vi "HS_EnableFrameBuffer.vi"(8 "error in":errorcluster, 9 "Console In":string, 11 "VISA Refnum in":refnum<visa-resource-name>) -> (0 "error out":errorcluster, 1 "Console Out":string, 2 "Reply":string, 3 "VISA Refnum out":refnum<visa-resource-name>)   [LabVIEW 2016]
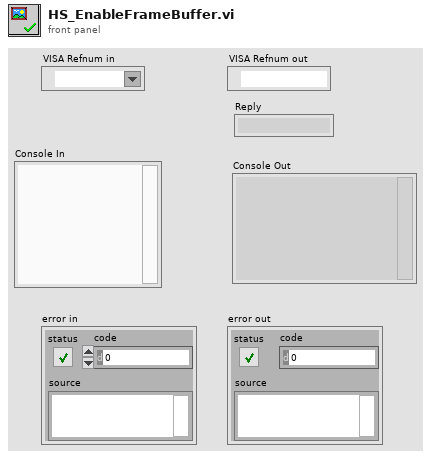
[diagram p1: front panel]
types:
  T1 = cluster{"Before":u8, "After":u8, "Send as 1 block?":bool}
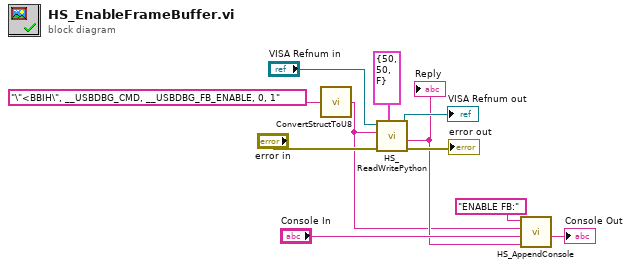
[diagram p0: block diagram]
diagram:
  n1 = call "ConvertStructToU8.vi"("struct"="\"<BBIH\", __USBDBG_CMD, __USBDBG_FB_ENABLE, 0, 1" ("write buffer")) -> ("Binary"=w2:string)
  n2 = call "HS_ReadWritePython.vi"("Timeouts (ms)"=T1 {"Before"=50, "After"=50, "Send as 1 block?"=FALSE}, "error in"="error in", "Write"=w2, "VISA in"="VISA Refnum in") -> ("error out"=→"error out":errorcluster, "Console Out"=w4:string, "VISA out"=→"VISA Refnum out":refnum<visa-resource-name>)  [unwired: 2 in, 3 out]
  "Reply" <- w4
  n3 = call "HS_AppendConsole.vi"("Reply"=w4, "Console in"="Console In", "Send"=w2, "Command"="ENABLE FB:") -> ("Console Out"=→"Console Out":string)  [unwired: 7 in]
